vi "NT Table Read Gyro.vi"() -> (3 "Gyro Angle (deg)":dbl)   [LabVIEW 2023]
uses:
  <vilib>/Rock Robotics/Network Tables/NT Read Number.vi
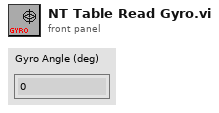
[diagram p1: front panel]
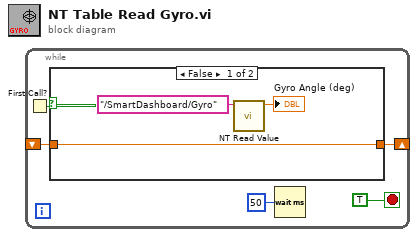
[diagram p0: block diagram]
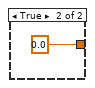
[diagram p2: hidden frame]
diagram:
  n1 = while {
    shift-right: [w4] -> _
    shift-left: _ -> [w3]
    stop <- TRUE stop-if-true
    n2 = First Call?() -> (First Call?: T/F=w5:bool)
    n3 = case shown="False" w5 {
      tunnel: [w7 0.0] -> w4
      tunnel: w3 -> [w7 _]
      frame False {
        n4 = call-poly <vilib>:"NT Read Value.vi"("name"="/SmartDashboard/Gyro" ("Name")) -> ("value"=→"Gyro Angle (deg)":dbl)  [unwired: 8 in, 2 out]
      }
      frame True {
      }
    }
    n5 = Wait (ms)(milliseconds to wait=u32 50) -> ()  [unwired: 1 out]
  }
